vi "TDC_DAQV16_after.vi"() -> ()   [LabVIEW 2017]
uses:
  <vilib>/Utility/file.llb/Write Delimited Spreadsheet (DBL).vi
  <vilib>/Utility/file.llb/Write Delimited Spreadsheet (I64).vi
panel:
  out "Array 5":u32[](array[numeric])=[0, 2, 4, 6, 8, 10, 12, 14, 0, 2, 4, 6, 8, 10, 12, 14, 0, 2, 4, 6, 8, 10, 12, 14, 0, 2, 4, 6, 8, 10, 12, 14] format="%x"
  out "Array 4":u32[](array[numeric])=[96, 96, 96, 96, 96, 96, 96, 96, 128, 128, 128, 128, 128, 128, 128, 128, 160, 160, 160, 160, 160, 160, 160, 160, 192, 192, 192, 192, 192, 192, 192, 192] format="%x"
  out "Array 3":u32[](array[numeric])=[0, 0, 0, 0, 0, 0, 0, 0, 32, 32, 32, 32, 32, 32, 32, 32, 64, 64, 64, 64, 64, 64, 64, 64, 96, 96, 96, 96, 96, 96, 96, 96] format="%x"
  out "Array 2":u32[](array[numeric])=[97, 99, 101, 103, 105, 107, 109, 111, 129, 131, 133, 135, 137, 139, 141, 143, 161, 163, 165, 167, 169, 171, 173, 175, 193, 195, 197, 199, 201, 203, 205, 207] format="%x"
  out "Array":u32[](array[numeric])=[96, 98, 100, 102, 104, 106, 108, 110, 128, 130, 132, 134, 136, 138, 140, 142, 160, 162, 164, 166, 168, 170, 172, 174, 192, 194, 196, 198, 200, 202, 204, 206] format="%x"
  in  "Thresholds (mV)":u16[](array[numeric])=[580, 540, 580, 580, 600, 600, 600, 600, 580, 580, 600, 600, 600, 600, 600, 600, 580, 580, 600, 600, 600, 600, 600, 600, 580, 580, 600, 600, 600, 600, 600, 600]
  in  "SMA mode":bool=TRUE
  out "error out 2":errorcluster={"status"=TRUE, "code"=1, "source"="Dequeue Element in TDC_DAQV16_after.vi"}
  in  "display":bool=TRUE
  in  "Thresholds":u16=600
  in  "one key for threshold":bool
  in  "save data":bool
  in  "RST":bool
  out "rate":dbl=1621.5429393180434
  out "appended path 2":path=path "G:/tdc/2017/test_20230924_115732.csv"
  in  "通道数量":i32=64
  out "Cal Table":u32[](array[numeric])=[5703, 5703, 5702, 5702, 0, 0, 0, 0, 0, 0, 0, 0, 0, 0, 0, 0, 0, 0, 0, 0, 0, 0, 0, 0, 0, 0, 0, 0, 0, 0, 0, 0, 0, 0, 0, 0, 0, 0, 0, 0, 0, 0, 0, 0, 0, 0, 0, 0, 0, 0, 0, 0, 0, 0, 0, 0, 0, 0, 0, 0, 0, 0, 0, 0]
  in  "channel for cal":i32=3
  out "single":u32 format="%08x"
  out "channel number":u64
  in  "bytes to read":i32=80
  out "Calibration Counter":i32=5702
  out "Event index":i32=97959
  out "cal":u32[](graph)=[0, 0, 0, 0, 0, 0, 0, 0, 0, 0, 0, 0, 0, 0, 0, 0, 0, 0, 0, 0, 0, 0, 0, 0, 0, 0, 0, 0, 0, 0, 0, 0, 0, 0, 0, 0, 0, 0, 0, 0, 0, 0, 0, 0, 0, 0, 0, 0, 0, 0, 0, 0, 0, 0, 0, 0, 0, 0, 0, 0, 0, 0, 0, 0, 0, 0, 0, 0, 0, 0, 0, 0, 0, 0, 0, 0, 0, 0, 0, 0, 0, 0, 0, 0, 0, 0, 0, 0, 0, 0, 0, 0, 0, 0, 0, 0, 0, 0, 0, 0, 0, 0, 0, 0, 0, 0, 0, 0, 0, 0, 0, 0, 0, 0, 0, 0, 0, 0, 0, 0, 0, 0, 0, 0, 0, 0, 0, 0, 0, 0, 0, 0, 0, 0, 0, 0, 0, 0, 0, 0, 0, 0, 0, 0, 0, 0, 0, 0, 0, 0, 0, 0, 0, 0, 0, 0, 0, 0, 0, 0, 0, 0, 0, 0, 0, 0, 0, 0, 0, 0, 0, 0, 0, 0, 0, 0, 0, 0, 0, 0, 0, 0, 0, 0, 0, 0, 0, 0, 0, 0, 0, 0, 0, 0, 0, 0, 0, 0, 0, 0, 0, 0, 0, 0, 0, 0, 0, 0, 0, 0, 0, 0, 0, 0, 0, 0, 0, 0, 0, 0, 0, 0, 0, 0, 0, 0, 0, 0, 0, 0, 0, 0, 0, 0, 0, 0, 0, 0, 0, 0, 0, 3, 5, 8, 9, 3, 11, 4, 12, 14, 15, 14, 41, 5, 29, 3, 6, 23, 3, 24, 19, 5, 24, 5, 4, 5, 8, 6, 8, 0, 3, 4, 3, 2, 5, 18, 13, 6, 2, 14, 0, 22, 1, 2, 15, 12, 3, 2, 32, 3, 6, 6, 8, 5, 16, 7, 19, 6, 3, 20, 11, 9, 17, 8, 23, 6, 7, 11, 6, 15, 2, 2, 15, 11, 3, 2, 10, 24, 10, 3, 4, 2, 1, 6, 1, 21, 10, 8, 0, 4, 4, 6, 4, 2, 8, 7, 17, 5, 5, 5, 1, 17, 4, 15, 9, 14, 16, 1, 8, 1, 1, 5, 18, 4, 3, 1, 11, 16, 1, 13, 8, 3, 0, 4, 29, 3, 10, 9, 3, 4, 12, 10, 8, 8, 3, 8, 14, 4, 16, 4, 7, 13, 7, 5, 17, 2, 4, 7, 9, 2, 4, 3, 2, 11, 4, 16, 9, 4, 6, 8, 2, 3, 12, 1, 24, 6, 5, 6, 17, 4, 6, 7, 6, 7, 3, 4, 4, 12, 8, 11, 3, 3, 17, 3, 6, 3, 10, 11, 15, 24, 10, 1, 2, 12, 14, 13, 30, 1, 3, 8, 14, 7, 21, 1, 5, 4, 1, 0, 7, 8, 13, 20, 6, 3, 3, 5, 1, 4, 11, 1, 2, 11, 6, 7, 5, 3, 2, 11, 3, 0, 2, 4, 7, 6, 12, 9, 12, 9, 6, 4, 6, 14, 6, 4, 2, 3, 35, 0, 4, 22, 2, 1, 23, 11, 43, 15, 10, 7, 3, 18, 3, 4, 25, 10, 9, 10, 11, 4, 4, 13, 16, 2, 1, 11, 11, 4, 2, 2, 5, 18, 3, 9, 11, 4, 4, 9, 3, 7, 10, 4, 2, 13, 5, 11, 13, 20, 5, 11, 9, 8, 5, 13, 27, 3, 15, 5, 4, 10, 13, 2, 6, 7, 3, 31, 6, 4, 9, 27, 4, 11, 3, 24, 2, 5, 3, 11, 2, 4, 3, 4, 10, 27, 9, 4, 3, 2, 1, 2, 1, 3, 1, 17, 3, 21, 1, 2, 2, 1, 14, 2, 33, 8, 20, 7, 8, 19, 4, 1, 10, 10, 3, 12, 6, 4, 4, 11, 2, 10, 5, 2, 6, 22, 10, 6, 2, 4, 6, 12, 8, 5, 3, 6, 11, 3, 11, 1, 14, 19, 4, 15, 1, 7, 6, 4, 5, 29, 3, 9, 3, 2, 5, 3, 6, 16, 5, 4, 16, 4, 0, 2, 1, 9, 8, 22, 2, 8, 6, 7, 2, 7, 1, 18, 4, 5, 10, 19, 6, 5, 5, 12, 4, 9, 12, 11, 2, 7, 9, 19, 1, 0, 27, 11, 11, 14, 4, 22, 6, 24, 7, 6, 14, 6, 34, 10, 4, 1, 1, 2, 1, 15, 10, 7, 8, 6, 4, 9, 2, 1, 2, 12, 7, 2, 4, 6, 3, 3, 4, 10, 8, 7, 5, 2, 30, 8, 18, 7, 3, 4, 23, 10, 33, 14, 4, 12, 4, 6, 5, 5, 16, 20, 7, 3, 4, 8, 5, 8, 16, 7, 31, 6, 2, 14, 5, 3, 6, 7, 15, 12, 11, 11, 4, 7, 9, 1, 8, 2, 7, 14, 2, 1, 8, 6, 1, 4, 1, 7, 4, 9, 13, 2, 3, 0, 1, 5, 11, 3, 3, 20, 14, 1, 17, 7, 8, 27, 14, 6, 3, 10, 13, 6, 15, 11, 5, 5, 11, 19, 3, 12, 14, 2, 4, 15, 12, 6, 9, 12, 4, 8, 4, 3, 14, 6, 5, 14, 0, 2, 1, 4, 21, 4, 23, 4, 0, 7, 4, 4, 3, 5, 24, 8, 4, 6, 11, 2, 8, 6, 6, 5, 22, 6, 6, 5, 4, 12, 30, 22, 1, 3, 11, 11, 15, 8, 5, 4, 3, 26, 2, 10, 19, 9, 10, 5, 12, 0, 8, 34, 7, 6, 30, 6, 13, 2, 5, 3, 29, 6, 5, 4, 10, 4, 2, 3, 3, 7, 11, 10, 3, 15, 4, 2, 1, 1, 15, 12, 7, 2, 2, 2, 12, 2, 19, 15, 16, 5, 3, 5, 7, 8, 4, 6, 25, 5, 5, 5, 7, 3, 7, 4, 4, 1, 1, 0, 0, 0, 0, 0, 0, 0, 0, 0, 0, 0, 0, 0, 0, 0, 0, 0, 0, 0, 0, 0, 0, 0, 0, 0, 0, 0, 0, 0, 0, 0, 0, 0, 0, 0, 0, 0, 0, 0, 0, 0, 0, 0, 0, 0, 0, 0, 0, 0, 0, 0, 0, 0, 0, 0, 0, 0, 0, 0, 0, 0, 0, 0, 0, 0, 0, 0, 0, 0, 0, 0, 0, 0, 0, 0, 0, 0, 0, 0, 0, 0, 0, 0, 0, 0, 0, 0, 0, 0, 0, 0, 0, 0, 0, 0, 0, 0, 0, 0, 0, 0, 0, 0, 0, 0, 0, 0, 0, 0, 0, 0, 0, 0, 0, 0, 0, 0, 0, 0, 0, 0, 0, 0, 0, 0, 0, 0, 0, 0, 0, 0, 0, 0, 0, 0, 0, 0, 0, 0, 0, 0, 0, 0, 0, 0, 0, 0, 0, 0, 0, 0, 0, 0, 0, 0, 0, 0, 0, 0, 0, 0, 0, 0, 0, 0, 0, 0, 0, 0, 0, 0, 0, 0, 0, 0, 0, 0, 0, 0, 0, 0, 0, 0, 0, 0, 0, 0, 0, 0, 0, 0, 0, 0, 0, 0, 0, 0, 0, 0, 0, 0, 0, 0, 0, 0, 0, 0, 0, 0, 0, 0, 0, 0, 0, 0, 0, 0, 0, 0, 0, 0, 0, 0, 0, 0, 0, 0, 0, 0, 0, 0, 0, 0, 0, 0, 0, 0, 0, 0, 0, 0, 0, 0, 0, 0, 0, 0, 0, 0, 0, 0, 0, 0, 0, 0, 0, 0, 0, 0, 0, 0, 0, 0, 0, 0, 0, 0, 0, 0, 0, 0, 0, 0, 0, 0, 0, 0, 0, 0, 0, 0, 0, 0, 0, 0, 0, 0, 0, 0, 0, 0, 0, 0, 0, 0, 0, 0, 0, 0, 0, 0, 0, 0, 0, 0, 0, 0, 0, 0, 0, 0, 0, 0, 0, 0, 0, 0, 0, 0, 0, 0, 0, 0, 0, 0, 0, 0, 0, 0, 0, 0, 0, 0, 0, 0, 0, 0, 0, 0, 0, 0, 0, 0, 0, 0, 0, 0, 0, 0, 0, 0, 0, 0, 0, 0, 0, 0, 0, 0, 0, 0, 0, 0, 0, 0, 0, 0, 0, 0, 0, 0, 0, 0, 0, 0, 0, 0, 0, 0, 0, 0, 0, 0, 0, 0, 0, 0, 0, 0, 0, 0, 0, 0, 0, 0, 0, 0, 0, 0, 0, 0, 0, 0, 0, 0, 0, 0, 0, 0, 0, 0, 0, 0, 0, 0, 0, 0, 0, 0, 0, 0, 0, 0, 0, 0, 0, 0, 0, 0, 0, 0, 0, 0, 0, 0, 0, 0, 0, 0, 0, 0, 0, 0, 0, 0, 0, 0, 0, 0, 0, 0, 0, 0, 0, 0, 0, 0, 0, 0, 0, 0, 0, 0, 0, 0, 0, 0, 0, 0, 0, 0, 0, 0, 0, 0, 0, 0, 0, 0, 0, 0, 0, 0, 0, 0, 0, 0, 0, 0, 0, 0, 0, 0, 0, 0, 0, 0, 0, 0, 0, 0, 0, 0, 0, 0, 0, 0, 0, 0, 0, 0, 0, 0, 0, 0, 0, 0, 0, 0, 0, 0, 0, 0, 0, 0, 0, 0, 0, 0, 0, 0, 0, 0, 0, 0, 0, 0, 0, 0, 0, 0, 0, 0, 0, 0, 0, 0, 0, 0, 0, 0, 0, 0, 0, 0, 0, 0, 0, 0, 0, 0, 0, 0, 0, 0, 0, 0, 0, 0, 0, 0, 0, 0, 0, 0, 0, 0, 0, 0, 0, 0, 0, 0, 0, 0, 0, 0, 0, 0, 0, 0, 0, 0, 0, 0, 0, 0, 0, 0, 0, 0, 0, 0, 0, 0, 0, 0, 0, 0, 0, 0, 0, 0, 0, 0, 0, 0, 0, 0, 0, 0, 0, 0, 0, 0, 0, 0, 0, 0, 0, 0, 0, 0, 0, 0, 0, 0, 0, 0, 0, 0, 0, 0, 0, 0, 0, 0, 0, 0, 0, 0, 0, 0, 0, 0, 0, 0, 0, 0, 0, 0, 0, 0, 0, 0, 0, 0, 0, 0, 0, 0, 0, 0, 0, 0, 0, 0, 0, 0, 0, 0, 0, 0, 0, 0, 0, 0, 0, 0, 0, 0, 0, 0, 0, 0, 0, 0, 0, 0, 0, 0, 0, 0, 0, 0, 0, 0, 0, 0, 0, 0, 0, 0, 0, 0, 0, 0, 0, 0, 0, 0, 0, 0, 0, 0, 0, 0, 0, 0, 0, 0, 0, 0, 0, 0, 0, 0, 0, 0, 0, 0, 0, 0, 0, 0, 0, 0, 0, 0, 0, 0, 0, 0, 0, 0, 0, 0, 0, 0, 0, 0, 0, 0, 0, 0, 0, 0, 0, 0, 0, 0, 0, 0, 0, 0, 0, 0, 0, 0, 0, 0, 0, 0, 0, 0, 0, 0, 0, 0, 0, 0, 0, 0, 0, 0, 0, 0, 0, 0, 0, 0, 0, 0, 0, 0, 0, 0, 0, 0, 0, 0, 0, 0, 0, 0, 0, 0, 0, 0, 0, 0, 0, 0, 0, 0, 0, 0, 0, 0, 0, 0, 0, 0, 0, 0, 0, 0, 0, 0, 0, 0, 0, 0, 0, 0, 0, 0, 0, 0, 0, 0, 0, 0, 0, 0, 0, 0, 0, 0, 0, 0, 0, 0, 0, 0, 0, 0, 0, 0, 0, 0, 0, 0, 0, 0, 0, 0, 0, 0, 0, 0, 0, 0, 0, 0, 0, 0, 0, 0, 0, 0, 0, 0, 0, 0, 0, 0, 0, 0, 0, 0, 0, 0, 0, 0, 0, 0, 0, 0, 0, 0, 0, 0, 0, 0, 0, 0, 0, 0, 0, 0, 0, 0, 0, 0, 0, 0, 0, 0, 0, 0, 0, 0, 0, 0, 0, 0, 0, 0, 0, 0, 0, 0, 0, 0, 0, 0, 0, 0, 0, 0, 0, 0, 0, 0, 0, 0, 0, 0, 0, 0, 0, 0, 0, 0, 0, 0, 0, 0, 0, 0, 0, 0, 0, 0, 0, 0, 0, 0, 0, 0, 0, 0, 0, 0, 0, 0, 0, 0, 0, 0, 0, 0, 0, 0, 0, 0, 0, 0, 0, 0, 0, 0, 0, 0, 0, 0, 0, 0, 0, 0, 0, 0, 0, 0, 0, 0, 0, 0, 0, 0, 0, 0, 0, 0, 0, 0, 0, 0, 0, 0, 0, 0, 0, 0, 0, 0, 0, 0, 0, 0, 0, 0, 0, 0, 0, 0, 0, 0, 0, 0, 0, 0, 0, 0, 0, 0, 0, 0, 0, 0, 0, 0, 0, 0, 0, 0, 0, 0, 0, 0, 0, 0, 0, 0, 0, 0, 0, 0, 0, 0, 0, 0, 0, 0, 0, 0, 0, 0, 0, 0, 0, 0, 0, 0, 0, 0, 0, 0, 0, 0, 0, 0, 0, 0, 0, 0, 0, 0, 0, 0, 0, 0, 0, 0, 0, 0]
  out "error out":errorcluster
  in  "stop":bool
  out "appended path":path=path "G:/tdc/2017/test_20230924_115732.dat"
  in  "filename":string="test"
  in  "Events":i32=110000 min=1
  in  "timeout (ms)":i32=10000
  in  "address":string="192.168.10.10"
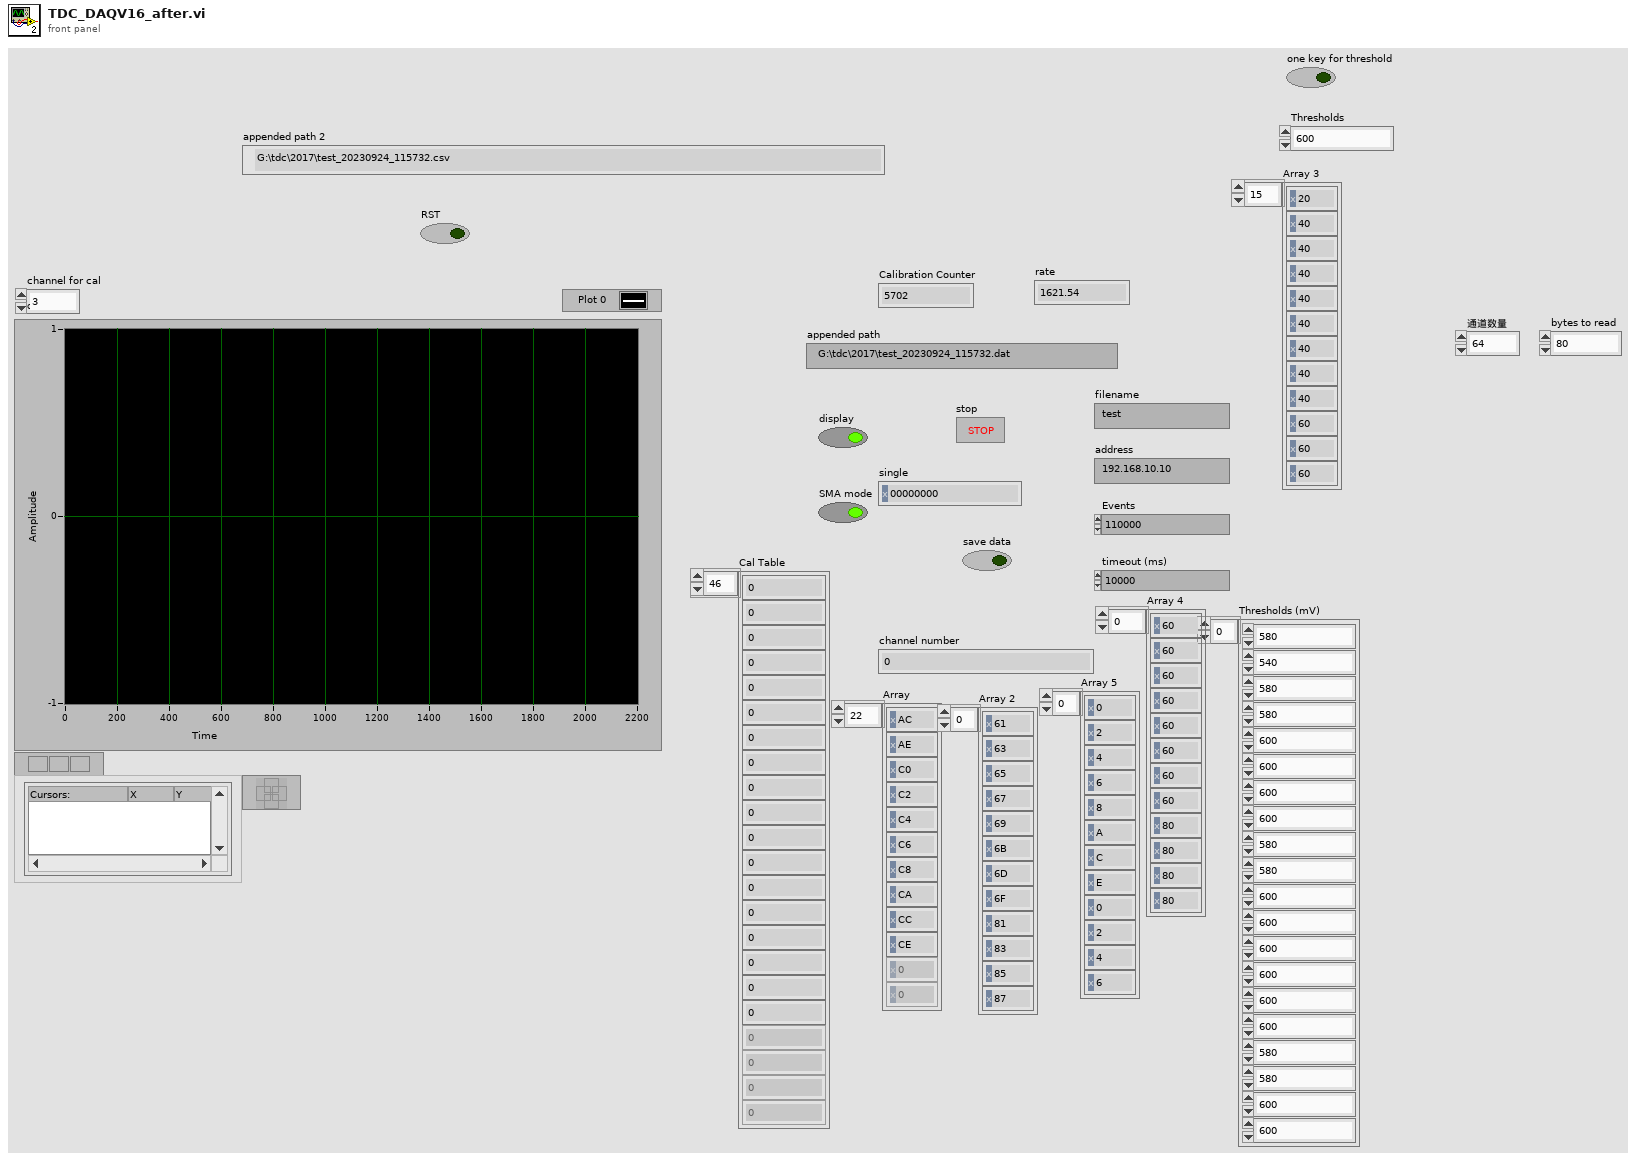
[diagram p1: front panel]
types:
  T1 = enum16{"open", "replace", "create", "open or create", "replace or create", "replace or create with confirmation"}
  T2 = enum16{"Standard", "Buffered", "CRLF", "Immediate"}
  T3 = enum16{"big-endian, network order", "native, host order", "little-endian"}
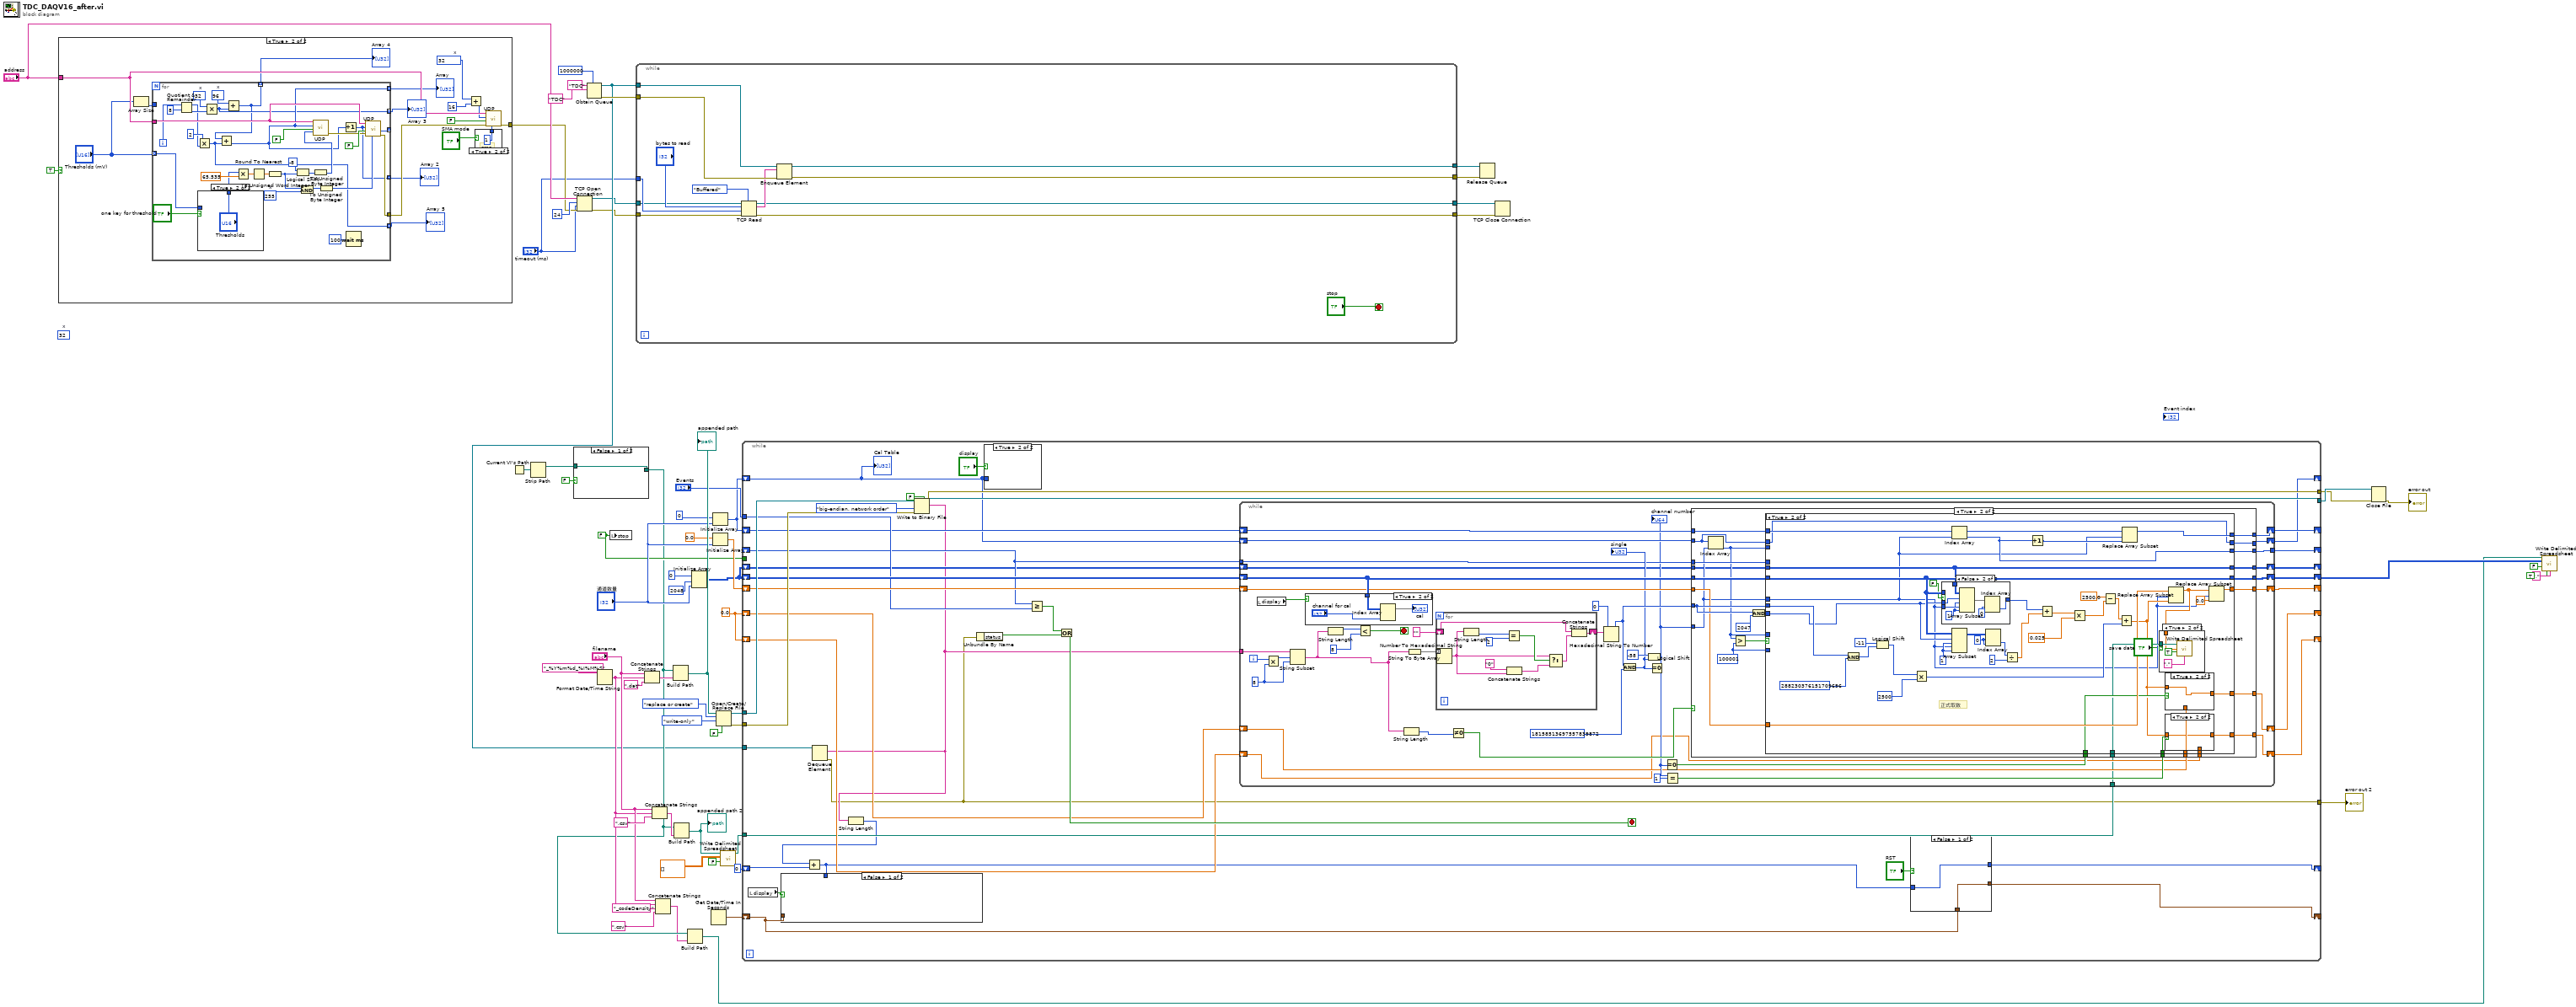
[diagram p0: block diagram]
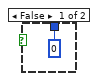
[diagram p3: hidden frame]
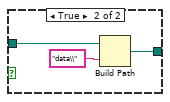
[diagram p5: hidden frame]
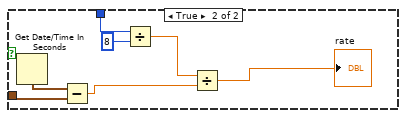
[diagram p6: hidden frame]
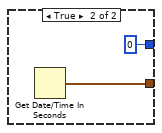
[diagram p8: hidden frame]
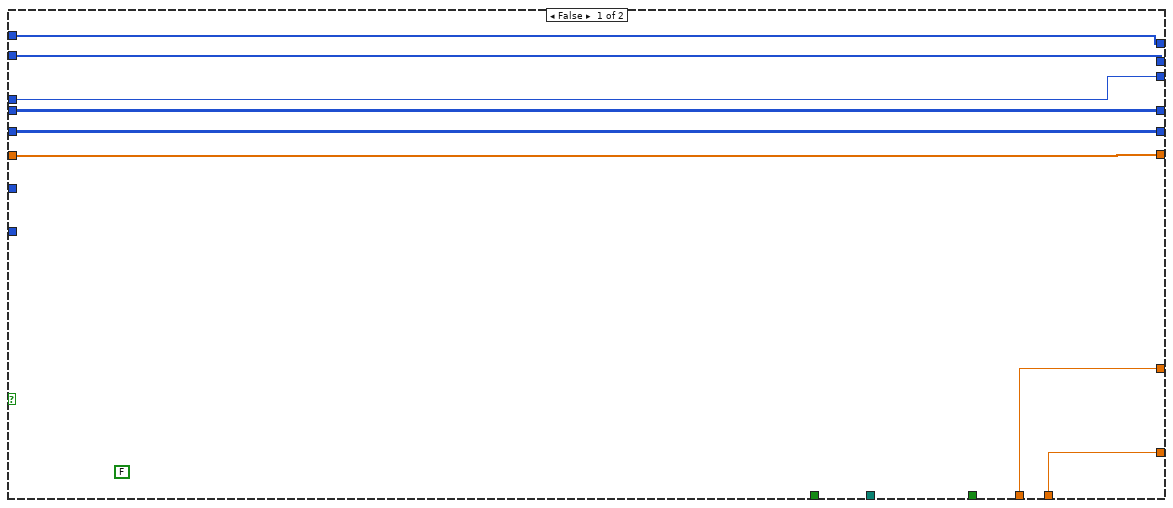
[diagram p10: hidden frame]
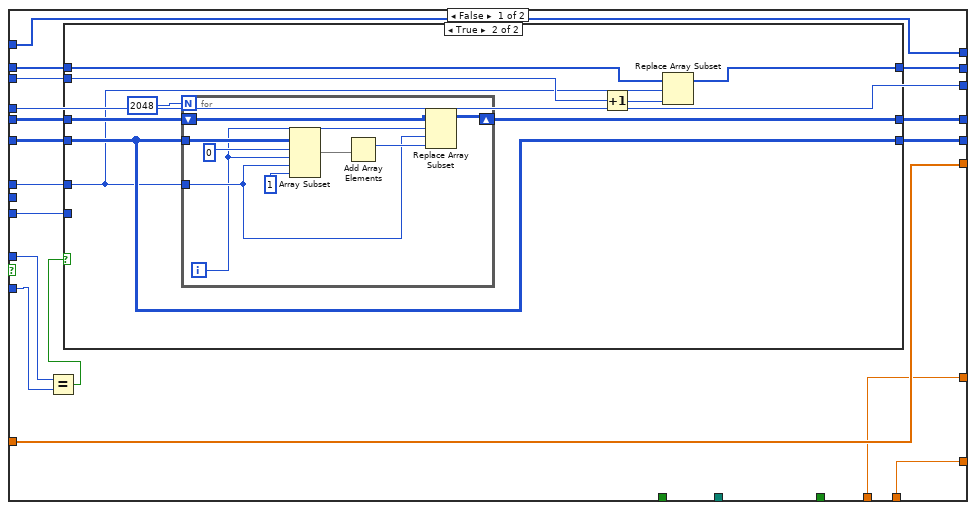
[diagram p11: hidden frame]
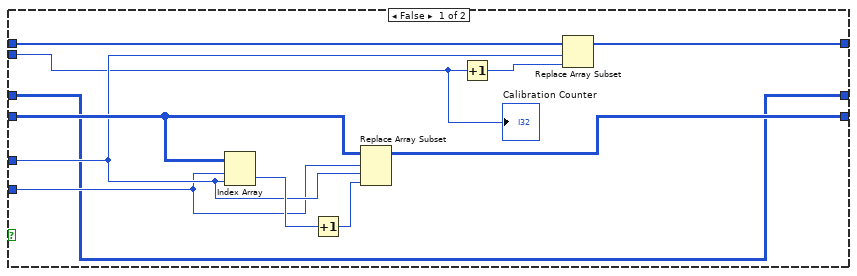
[diagram p12: hidden frame]
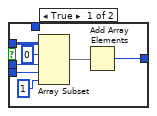
[diagram p14: hidden frame]
diagram:
  (unwired) u16 32  # x
  w26 = FALSE ("stop")
  w38 = 0.0
  n1 = case shown="True" TRUE {
    tunnel: "address" -> [_ w78]
    tunnel: [_ w75] -> w27
    frame False {
    }
    frame True {
      w64 = u16 32  # x
      n2 = Array Size(array="Thresholds (mV)") -> (size(s)=w72:i32)
      n3 = for {
        tunnel: w78 -> [w107]
        tunnel: "Thresholds (mV)" -> [w93] mode=indexing
        tunnel: [w101] -> _ mode=indexing
        tunnel: [w96] -> w76
        tunnel: w72 -> [_]
        tunnel: [w87] -> w70 mode=indexing
        tunnel: [w86] -> w69 mode=indexing
        tunnel: [w85] -> w68 mode=indexing
        tunnel: [w84] -> w67 mode=indexing
        tunnel: [w83] -> w66 mode=indexing
        i -> [w88]
        w89 = u16 96  # x
        w90 = u16 32  # x
        w103 = u16 255  # x
        n4 = Quotient & Remainder(x=w88, y=8) -> (x-y*floor(x/y)=w82:i32, floor(x/y)=w91:i32)
        n5 = Multiply(x=2, y=w82) -> (x*y=w83:i32)
        n6 = case shown="True" "one key for threshold" {
          tunnel: [w113 "Thresholds"] -> w94
          tunnel: w93 -> [w113 _]
          frame False {
          }
          frame True {
          }
        }
        n7 = Multiply(x=w90, y=w91) -> (x*y=w85:i32)
        n8 = Add(x=w89, y=w85) -> (x+y=w84:i32)
        n9 = Add(x=w84, y=w83) -> (x+y=w87:i32)
        n10 = Multiply(x=w94, y=65.535) -> (x*y=w110:dbl)
        n11 = Round To Nearest(number=w110) -> (nearest integer value=w108:dbl)
        n12 = To Unsigned Word Integer(number=w108) -> (unsigned 16bit integer=w98:u16)
        n13 = Logical Shift(y=i16 -8, x=w98) -> (x << y=w105:u16)
        n14 = And(x=w98, y=w103) -> (x .and. y?=w102:u16)
        n15 = To Unsigned Byte Integer(number=w105) -> (unsigned 8bit integer=w104:u8)
        n16 = call "UDP.vi"("In"=w104, "Read (TRUE)"=FALSE, "Address"=w87, "IP address"=w107) -> ("error out"=w97:errorcluster)  [unwired: 5 in, 1 out]
        n17 = To Unsigned Byte Integer(number=w102) -> (unsigned 8bit integer=w100:u8)
        n18 = Increment(x=w87) -> (x+1=w86:i32)
        n19 = Wait (ms)(milliseconds to wait=u32 100) -> ()  [unwired: 1 out]
        n20 = call "UDP.vi"("In"=w100, "error in (no error)"=w97, "Read (TRUE)"=FALSE, "Address"=w86, "IP address"=w107) -> ("error out"=w96:errorcluster, "Out"=w101:u8)  [unwired: 4 in]
      }
      "Array" <- w70
      "Array 2" <- w69
      "Array 3" <- w68
      "Array 4" <- w67
      "Array 5" <- w66
      n21 = Add(x=w64, y=u32 16 ("Address")) -> (x+y=w63:u32)
      n22 = case shown="True" "SMA mode" {
        tunnel: [u8 0 ("In") u8 1 ("In")] -> w74
        frame False {
        }
        frame True {
          # "sma"
        }
      }
      n23 = call "UDP.vi"("In"=w74, "error in (no error)"=w76, "Read (TRUE)"=FALSE, "Address"=w63, "IP address"=w78) -> ("error out"=w75:errorcluster)  [unwired: 4 in, 1 out]
    }
  }
  n24 = Current VI's Path() -> (path=w56:path)
  n25 = Strip Path(path=w56) -> (stripped path=w55:path)  [unwired: 1 out]
  n26 = case shown="False" FALSE {
    tunnel: w55 -> [w115 w117]
    tunnel: [w115 w116] -> w21
    frame False {
    }
    frame True {
      n27 = Build Path(base path=w117, name or relative path="data\\") -> (appended path=w116:path)
    }
  }
  n28 = TCP Open Connection(address="address", remote port or service name=u16 24 ("port"), timeout ms (60000)="timeout (ms)", error in (no error)=w27) -> (connection ID=w9:refnum<k5>, error out=w10:errorcluster)  [unwired: 1 in]
  n29 = Obtain Queue(max queue size (-1, unlimited)=1000000, name (unnamed)="TDC", element data type="TDC" ("name (unnamed)")) -> (queue out=w11:refnum<queue>, error out=w12:errorcluster)  [unwired: 2 in, 1 out]
  n30 = Format Date/Time String(time format string (%c)="_%Y%m%d_%I%M%S") -> (date/time string=w24:string)  [unwired: 2 in]
  n31 = local write "stop"(w26) -> ()
  n32 = while {
    tunnel: w11 -> [w131]
    tunnel: w12 -> [w130]
    tunnel: w10 -> [w128]
    tunnel: "timeout (ms)" -> [w127]
    tunnel: w9 -> [w126]
    tunnel: [w124] -> w8
    tunnel: [w123] -> w7
    tunnel: [w121] -> w6
    tunnel: [w120] -> w5
    stop <- "stop" stop-if-true
    n33 = TCP Read(connection ID=w126, bytes to read="bytes to read", error in (no error)=w128, 7:T2."Buffered" ("mode (standard)"), 9:w127) -> (connection ID out=w124:refnum<k5>, data out=w125:string, error out=w123:errorcluster)
    n34 = Enqueue Element(queue=w131, element=w125, error in (no error)=w130) -> (queue out=w121:refnum<queue>, error out=w120:errorcluster)  [unwired: 1 in, 1 out]
  }
  n35 = Concatenate Strings("filename", w24, ".dat") -> (w54:string)
  n36 = Concatenate Strings("filename", w24, ".csv") -> (w40:string)
  n37 = Concatenate Strings("filename", w24, "_codeDensity" ("string"), ".csv") -> (w20:string)
  n38 = Build Path(base path=w21, name or relative path=w54) -> (appended path=w53:path)
  "appended path" <- w53
  n39 = Build Path(base path=w21, name or relative path=w40) -> (appended path=w35:path)
  "appended path 2" <- w35
  n40 = Build Path(base path=w21, name or relative path=w20) -> (appended path=w17:path)
  n41 = Initialize Array(u32 0 ("element"), 2048 ("dimension size"), "通道数量") -> (w37:u32[][])
  n42 = Get Date/Time In Seconds() -> (seconds since 1Jan1904=w29:timestamp)
  n43 = Initialize Array(u32 0 ("element"), "通道数量") -> (w39:u32[])
  n44 = Initialize Array(0.0, "通道数量") -> (w45:dbl[])
  n45 = Open/Create/Replace File(file path (use dialog)=w53, operation (0:open)=T1."replace or create", access (0:read/write)=enum16{"read/write", "read-only", "write-only"}."write-only", disable buffering (F)=FALSE) -> (refnum out=w58:refnum<file>, error out=w57:errorcluster)  [unwired: 2 in, 1 out]
  n46 = call-poly <vilib>:"Write Delimited Spreadsheet.vi"("file path (dialog if empty)"=w35, "2D data"=dbl[][] [], "append to file? (new file:F)"=FALSE) -> ("new file path (Not A Path if cancelled)"=w34:path)  [unwired: 11 in, 1 out]
  n47 = while {
    tunnel: w58 -> [w169]
    tunnel: w57 -> [w170]
    tunnel: [w133] -> w4
    tunnel: [w168] -> w50
    tunnel: [w167] -> w49
    shift-right: [w163] -> w18
    shift-left: w37 -> [w164]
    shift-right: [w147] -> _
    shift-left: w45 -> [w162]
    tunnel: "Events" -> [w159]
    shift-right: [w158] -> _
    shift-left: w39 -> [w157]
    shift-right: [w156] -> _
    shift-left: _ -> [w155]
    shift-right: [w154] -> _
    shift-left: w39 -> [w136]
    shift-right: [w153] -> _
    shift-left: w38 -> [w150]
    shift-right: [w152] -> _
    shift-left: w38 -> [w151]
    shift-right: [w139] -> _
    shift-left: w37 -> [w149]
    tunnel: w34 -> [w148]
    shift-right: [w143] -> _
    shift-left: 0 -> [w146]
    shift-right: [w141] -> _
    shift-left: w29 -> [w140]
    tunnel: w26 -> [_]
    tunnel: w11 -> [w135]
    stop <- w161 stop-if-true
    n48 = local read "display"() -> (w137:bool)
    n49 = Dequeue Element(queue=w135) -> (element=w134:string, error out=w133:errorcluster)  [unwired: 2 in, 2 out]
    n50 = String Length(string=w134) -> (length=w145:i32)
    n51 = Add(x=w145, y=w146) -> (x+y=w144:i32)
    n52 = case shown="False" w137 {
      tunnel: w144 -> [_ w172]
      tunnel: w140 -> [_ w171]
      frame False {
      }
      frame True {
        n53 = Get Date/Time In Seconds() -> (seconds since 1Jan1904=w176:timestamp)
        n54 = Subtract(x=w176, y=w171) -> (x-y=w175:dbl)
        n55 = Divide(x=w172, y=8) -> (x/y=w174:dbl)
        n56 = Divide(x=w174, y=w175) -> (x/y=→"rate":dbl)
      }
    }
    n57 = Write to Binary File(file (use dialog)=w169, data=w134, error in=w170, 5:FALSE ("prepend array or string size? (T)"), 9:T3."big-endian, network order" ("byte order (0:big-endian, network order)")) -> (refnum out=w168:refnum<file>, error out=w167:errorcluster)  [unwired: 1 in, 1 out]
    n58 = Unbundle By Name(w133) -> ("status"=w132:bool)
    n59 = case shown="True" "display" {
      tunnel: w136 -> [_ _]
      frame False {
      }
      frame True {
      }
    }
    n60 = Greater Or Equal?(x=w155, y=w159) -> (x >= y?=w160:bool)
    n61 = Or(x=w160, y=w132) -> (x .or. y?=w161:bool)
    n62 = while {
      tunnel: w134 -> [w217]
      shift-right: [w213] -> w163
      shift-left: w164 -> [w211]
      shift-right: [w209] -> w147
      shift-left: w162 -> [w210]
      shift-right: [w203] -> w158
      shift-left: w157 -> [w202]
      tunnel: [w201] -> w156
      tunnel: w155 -> [w200]
      shift-right: [w198] -> w154
      shift-left: w136 -> [w199]
      shift-right: [w190] -> w153
      shift-left: w150 -> [w188]
      shift-right: [w186] -> w152
      shift-left: w151 -> [w187]
      tunnel: w148 -> [w184]
      shift-right: [w183] -> w139
      shift-left: w149 -> [w185]
      i -> [w215]
      stop <- w206 stop-if-true
      w214 = 8 ("length (rest)")
      n63 = local read "display"() -> (w182:bool)
      n64 = Multiply(x=w215, y=w214) -> (x*y=w216:i32)
      n65 = String Subset(string=w217, offset (0)=w216, length (rest)=w214) -> (substring=w197:string)
      n66 = case shown="True" w182 {
        tunnel: w211 -> [_ w224]
        frame False {
        }
        frame True {
          n67 = Index Array(array=w224, index (col)="channel for cal") -> (element=→"cal":u32[])  [unwired: 1 in]
        }
      }
      n68 = String Length(string=w197) -> (length=w208:i32)
      n69 = Less?(x=w208, y=8) -> (x < y?=w206:bool)
      n70 = String Length(string=w197) -> (length=w195:i32)
      n71 = String To Byte Array(string=w197) -> (unsigned byte array=w220:u8[])
      n72 = for {
        shift-right: [w377] -> w219
        shift-left: "" ("format string") -> [w374]
        tunnel: w220 -> [w378] mode=indexing
        n73 = Number To Hexadecimal String(2:w378) -> (0:w370:string)  [unwired: 1 in]
        n74 = String Length(string=w370) -> (length=w376:i32)
        n75 = Equal?(x=w376, y=2) -> (x = y?=w373:bool)
        n76 = Concatenate Strings("0" ("format string"), w370) -> (w372:string)
        n77 = Select(t=w370, s=w373, f=w372) -> (s? t:f=w369:string)
        n78 = Concatenate Strings(w374, w369) -> (w377:string)
      }
      n79 = Not Equal To 0?(x=w195) -> (x != 0?=w194:bool)
      n80 = Hexadecimal String To Number(string=w219, default (0uL)=u64 0 ("default (0 U32)")) -> (number=w212:u64)  [unwired: 1 in, 1 out]
      n81 = And(x=w212, y=u64 18158513697557839872 ("port")) -> (x .and. y?=w204:u64)
      "single" <- w204
      n82 = Logical Shift(y=i16 -58, x=w204) -> (x << y=w193:u64)
      "channel number" <- w193
      n83 = Equal To 0?(x=w204) -> ()  [unwired: 1 out]
      n84 = Equal To 0?(x=w193) -> (x = 0?=w191:bool)
      n85 = Equal?(x=w193, y=u64 1) -> (x = y?=w189:bool)
      n86 = case shown="True" w194 {
        tunnel: w212 -> [_ w258]
        tunnel: w200 -> [w229 w248]
        tunnel: w211 -> [w232 w257]
        tunnel: [w232 w256] -> w213
        tunnel: [w231 w253] -> w209
        tunnel: w210 -> [w231 w252]
        tunnel: w193 -> [_ w247]
        tunnel: w202 -> [w230 w251]
        tunnel: [w230 w250] -> w203
        tunnel: [w229 w249] -> w201
        tunnel: w199 -> [w228 w246]
        tunnel: [w228 w245] -> w198
        tunnel: w191 -> [_ w244]
        tunnel: w188 -> [w227 w243]
        tunnel: [w227 w242] -> w190
        tunnel: w189 -> [_ w241]
        tunnel: w187 -> [w226 w240]
        tunnel: [w226 w239] -> w186
        tunnel: w185 -> [w225 w236]
        tunnel: [w225 w235] -> w183
        tunnel: w184 -> [_ w234]
        frame False {
          (unwired) FALSE
        }
        frame True {
          w237 = 100001 ("y")
          n87 = Index Array(array=w246, index=w247) -> (element=w238:u32)
          n88 = Greater?(x=w238, y=w237) -> (0:w233:bool)
          n89 = And(x=w258, y=u64 2047 ("port")) -> (x .and. y?=w254:u64)
          n90 = case shown="True" w233 {
            tunnel: w258 -> [_ w346]
            tunnel: w257 -> [w275 w328]
            tunnel: [w274 w328] -> w256
            tunnel: w254 -> [w266 w326]
            tunnel: [w273 w309] -> w253
            tunnel: w252 -> [w273 w335]
            tunnel: w248 -> [w271 _]
            tunnel: w247 -> [w269 w307]
            tunnel: w251 -> [w272 w334]
            tunnel: [w272 w333] -> w250
            tunnel: [w271 w331] -> w249
            tunnel: w238 -> [w267 _]
            tunnel: w246 -> [w270 w330]
            tunnel: [w268 w330] -> w245
            tunnel: w244 -> [_ w322]
            tunnel: w243 -> [w265 w321]
            tunnel: [w265 w320] -> w242
            tunnel: w241 -> [_ w319]
            tunnel: w240 -> [w264 w318]
            tunnel: [w264 w317] -> w239
            tunnel: w238 -> [w262 _]
            tunnel: w237 -> [w259 _]
            tunnel: w236 -> [w261 w311]
            tunnel: [w260 w311] -> w235
            tunnel: w234 -> [_ w310]
            frame False {
              n91 = Equal?(x=w262, y=w259) -> (x = y?=w263:bool)
              n92 = case shown="True" w263 {
                tunnel: w275 -> [w286 w292]
                tunnel: [w284 w292] -> w274
                tunnel: w270 -> [w282 w290]
                tunnel: w269 -> [w281 w287]
                tunnel: [w279 w289] -> w268
                tunnel: w267 -> [w278 w288]
                tunnel: w266 -> [w277 _]
                tunnel: w261 -> [w276 w294]
                tunnel: [w276 w293] -> w260
                frame False {
                  n93 = Index Array(array=w286, index (row)=w277, index (col)=w281) -> (element=w285:u32)
                  n94 = Increment(x=w285) -> (x+1=w283:u32)
                  n95 = Replace Array Subset(array=w286, new element=w283, index (row)=w277, index (col)=w281) -> (w284:u32[][])
                  n96 = Increment(x=w278) -> (x+1=w280:u32)
                  n97 = Replace Array Subset(array=w282, new element=w280, index=w281) -> (w279:u32[])
                  "Calibration Counter" <- w278
                }
                frame True {
                  n98 = for {
                    N: 2048 -> [_]
                    tunnel: w292 -> [w304]
                    tunnel: w287 -> [w297]
                    shift-right: [w299] -> w293
                    shift-left: w294 -> [w300]
                    i -> [w296]
                    n99 = Array Subset(array=w304, index (row)=0 ("索引"), length (row)=w296, index (col)=w297, length (col)=1 ("长度")) -> (w301:u32[][])
                    n100 = Add Array Elements(numeric array=w301) -> (sum=w298:u32)
                    n101 = Replace Array Subset(array=w300, new element=w298, index (row)=w296, index (col)=w297) -> (w299:u32[][])
                  }
                  n102 = Increment(x=w288) -> (x+1=w291:u32)
                  n103 = Replace Array Subset(array=w290, new element=w291, index=w287) -> (w289:u32[])
                }
              }
            }
            frame True {
              w324 = 0 ("索引 (行)")
              w327 = 1 ("长度")
              # "正式取数"
              n104 = And(x=w346, y=u64 288230376151709696 ("port")) -> (x .and. y?=w343:u64)
              n105 = Logical Shift(y=i16 -11, x=w343) -> (x << y=w338:u64)
              n106 = Multiply(x=w338, y=u64 2500) -> (x*y=w336:u64)
              n107 = case shown="False" FALSE {
                tunnel: [w352 w359] -> w341
                tunnel: w328 -> [w355 _]
                tunnel: w307 -> [w354 w364]
                tunnel: w326 -> [w353 w362]
                tunnel: w311 -> [_ w363]
                frame True {
                  n108 = Array Subset(array=w355, index (row)=0 ("索引"), length (row)=w353, index (col)=w354, length (col)=1 ("长度")) -> (w356:u32[][])
                  n109 = Add Array Elements(numeric array=w356) -> (sum=w352:u32)
                }
                frame False {
                  w358 = 0 ("index (row)")
                  w361 = 1 ("长度")
                  n110 = Array Subset(array=w363, index (row)=w362, length (row)=w361, index (col)=w364, length (col)=w361) -> (w360:u32[][])
                  n111 = Index Array(array=w360, index (row)=w358, index (col)=w358) -> (element=w359:u32)
                }
              }
              n112 = Index Array(array=w334, index=w307) -> (element=w331:u32)
              n113 = Array Subset(array=w328, index (row)=w326, length (row)=w327, index (col)=w307, length (col)=w327) -> (w325:u32[][])
              n114 = Index Array(array=w325, index (row)=w324, index (col)=w324) -> (element=w323:u32)
              n115 = Divide(x=w323, y=u32 2) -> (x/y=w329:dbl)
              n116 = Increment(x=w331) -> (x+1=w332:u32)
              n117 = Add(x=w341, y=w329) -> (x+y=w340:dbl)
              n118 = Multiply(x=w340, y=0.025) -> (x*y=w314:dbl)
              n119 = Subtract(x=2500.0, y=w314) -> (x-y=w313:dbl)
              n120 = Add(x=w313, y=w336) -> (x+y=w316:dbl)
              n121 = Replace Array Subset(array=w334, new element=w332, index=w307) -> (w333:u32[])
              n122 = case shown="True" w322 {
                tunnel: w316 -> [_ w368]
                tunnel: [w367 w368] -> w320
                tunnel: w321 -> [w367 _]
                frame False {
                }
                frame True {
                }
              }
              n123 = case shown="True" w319 {
                tunnel: [w365 w366] -> w317
                tunnel: w318 -> [w365 _]
                tunnel: w316 -> [_ w366]
                frame False {
                }
                frame True {
                }
              }
              n124 = Replace Array Subset(array=w335, new element=w316, index=w307) -> (w308:dbl[])
              n125 = case shown="True" "save data" {
                tunnel: w310 -> [_ w350]
                tunnel: w308 -> [_ w347]
                frame False {
                }
                frame True {
                  n126 = call-poly <vilib>:"Write Delimited Spreadsheet.vi"("file path (dialog if empty)"=w350, "1D data"=w347, "append to file? (new file:F)"=TRUE, "delimiter (\\t)"="," ("delimiter (\\t)")) -> ()  [unwired: 10 in, 2 out]
                }
              }
              n127 = Replace Array Subset(array=w308, new element=0.0 ("new element/subarray"), index=w307) -> (w309:dbl[])
            }
          }
        }
      }
    }
    n128 = case shown="False" "RST" {
      tunnel: w144 -> [w179 _]
      tunnel: [w179 0] -> w143
      tunnel: [w178 w180] -> w141
      tunnel: w140 -> [w178 _]
      frame False {
      }
      frame True {
        n129 = Get Date/Time In Seconds() -> (seconds since 1Jan1904=w180:timestamp)
      }
    }
    "Cal Table" <- w136
  }
  "error out 2" <- w4
  n130 = Release Queue(queue=w6, error in (no error)=w5) -> ()  [unwired: 1 in, 3 out]
  n131 = TCP Close Connection(connection ID=w8, error in (no error)=w7) -> ()  [unwired: 1 in, 2 out]
  n132 = Close File(refnum=w50, error in=w49) -> (error out=→"error out":errorcluster)  [unwired: 1 out]
  n133 = call-poly <vilib>:"Write Delimited Spreadsheet.vi"("file path (dialog if empty)"=w17, "2D data"=w18, "append to file? (new file:F)"=FALSE, "transpose? (no:F)"=TRUE, "delimiter (\\t)"="," ("delimiter (\\t)")) -> ()  [unwired: 9 in, 2 out]
